vi "Main Page.vi"(8 "error in (no error)":errorcluster, 11 "Node Ptr":T3 format="%.0x") -> (0 "error out":errorcluster)   [LabVIEW 2023, in "Embedded TDMS Logger System Explorer.lvlib"]
uses:
  Embedded TDMS Logger System Explorer.lvlib
  <vilib>/NI VeriStand/Custom Device API/Custom Device Item Ref.ctl
  Shared/SegmentOptions.ctl
  <vilib>/NI VeriStand/Custom Device API/Custom Device Channel.ctl
  <vilib>/NI VeriStand/Custom Device API/Custom Device Channel Type.ctl
  Shared/Meta Data Item.ctl
  <vilib>/NI VeriStand/Custom Device API/Get Item Property (U16).vi
  <vilib>/NI VeriStand/Custom Device API/Get Item Property (String).vi
  <vilib>/NI VeriStand/Custom Device API/Set Item Property (String).vi
  <vilib>/NI VeriStand/Custom Device API/Set Item Property (U16).vi
  <vilib>/NI VeriStand/Custom Device API/Get Item Property (Variant).vi
  <vilib>/NI VeriStand/Custom Device API/Set Item Property (Variant).vi
  <vilib>/NI VeriStand/Custom Device API/Set Item Property (Boolean).vi
  <vilib>/NI VeriStand/Custom Device API/Set Item Property (U64).vi
  <vilib>/NI VeriStand/Custom Device API/Custom Device API.lvlib
  Shared/Embedded TDMS Logger Shared.lvlib
panel:
  in  "Tab Control":T1(tab)
  out "String 3":string="The data format can be specified in the string, as with the formats specified in: https://www.ni.com/docs/en-US/bundle/labview-api-ref/page/functions/format-date-time-string.html"
  in  "Segment every":dbl=3600.0
  in  "Segment by":T2=enum."Size (MB)"
  in  "Filename Format:":string="mytestfile_%Y-%M-%d-%H-%I-%S.tdms"
  in  "Log Directory":path=path "c:/nirt/veristand/logs"
  in  "Segment Files":bool=TRUE
  out "String":string="Unless set, the system will trigger immediately to log upon deployment. If triggering is however enabled the log will start when the trigger channel receives a non-zero value. It will only stop logging once the system is undeployed."
  in  "Start on Trigger":bool
  in  "File Level Meta Data":string[][](table)=[["Software Version"], ["Test Rig Used"], ["UUT"], ["Operator"]]
  in  "Async Timeout (ms)":u16
  out "Version":string
  in  "Specific Header":cluster{"Section Name":string}={"Section Name"="Custom Device Item Settings"}
  in  "General Header":cluster{"Section Name":string}={"Section Name"="General Custom Device Settings"}
  in  "Description":string
  in  "Name":string
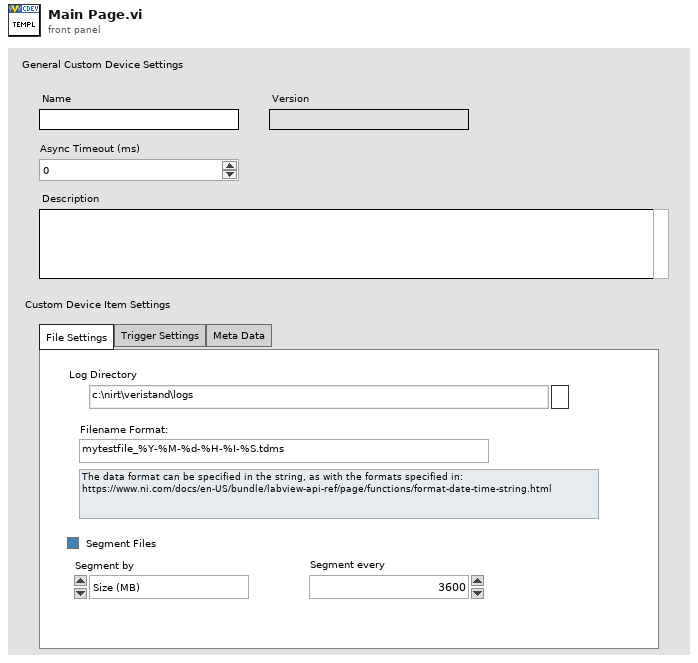
[diagram p1: front panel]
types:
  T1 = enum32{"File Settings", "Trigger Settings", "Meta Data"}
  T2 = typedef "SegmentOptions.ctl" = enum16{"Time (s)", "Size (MB)"}
  T3 = typedef "Custom Device API.lvlib/Custom Device Item Ref.ctl" = u64
  T4 = typedef "Custom Device API.lvlib/Custom Device Channel.ctl" = cluster{"Type":T5, "Units":string, "Default Value":dbl, "Faultable":bool, "Scalable":bool}
  T5 = typedef "Custom Device API.lvlib/Custom Device Channel Type.ctl" = enum16{"Input", "Output"}
  T6 = typedef "Custom Device API.lvlib/Custom Device Item Info.ctl" = cluster{"Name":string, "Is Channel":bool, "GUID":string, "Is Waveform":bool}
  T7 = typedef "Embedded TDMS Logger Shared.lvlib/Meta Data Item.ctl" = cluster{"Key":string, "Value":string}
  T8 = typedef "Custom Device API.lvlib/Custom Device Commands.ctl" = enum16{"Default", "Item renamed", "Shutdown", "Dynamic button pressed"}
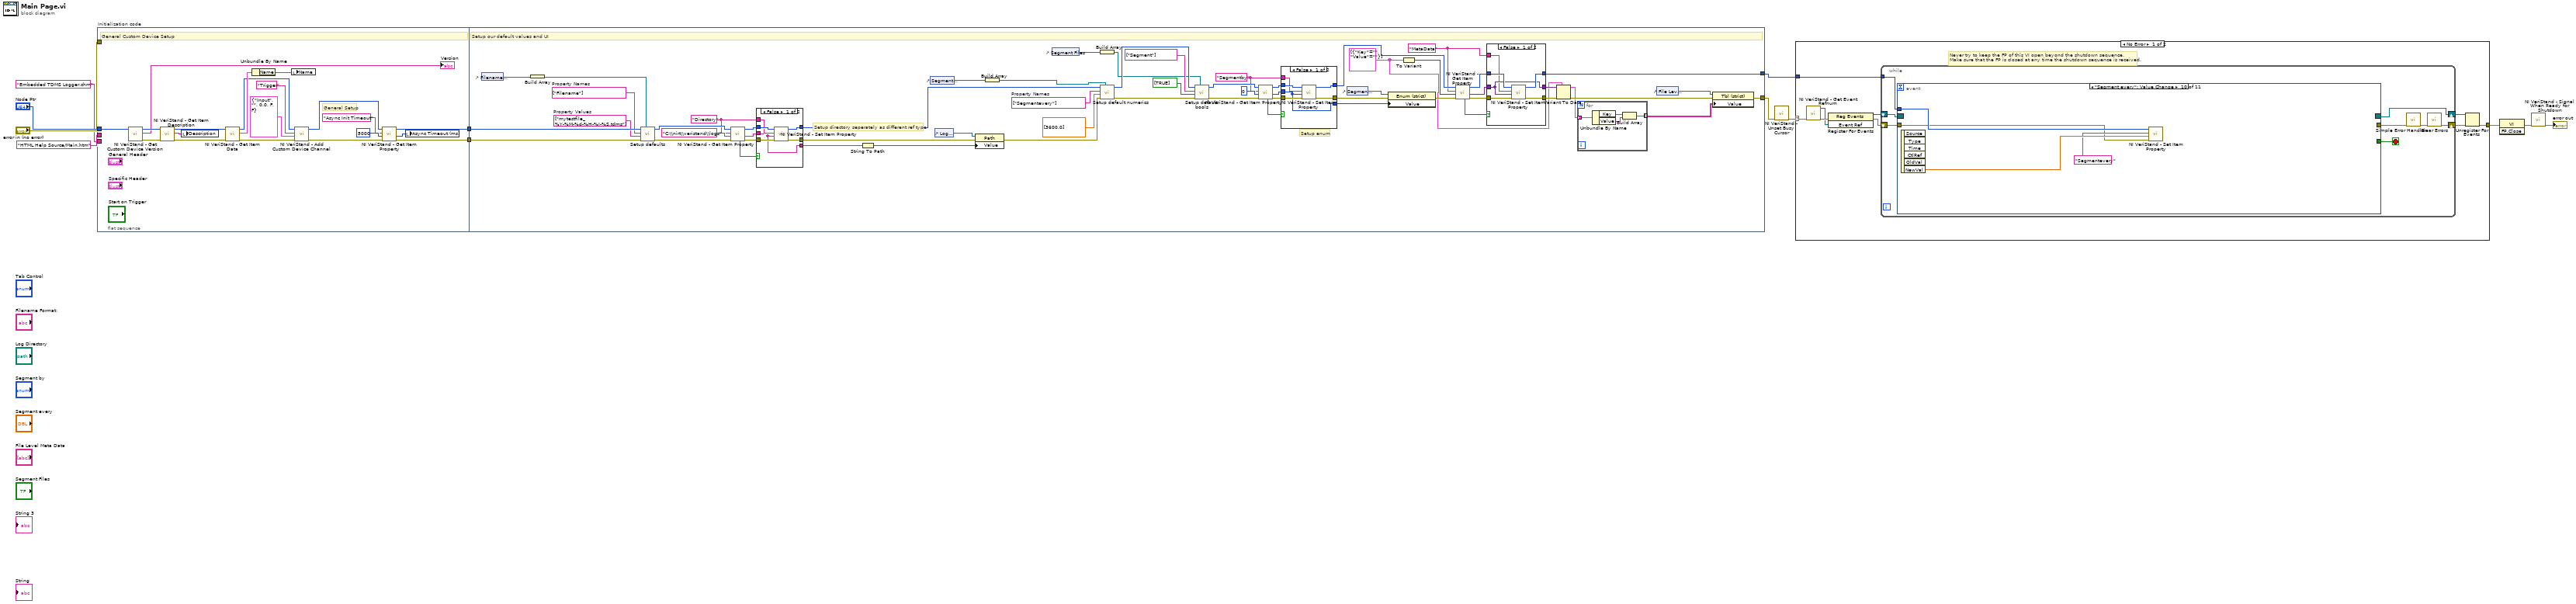
[diagram p0: block diagram]
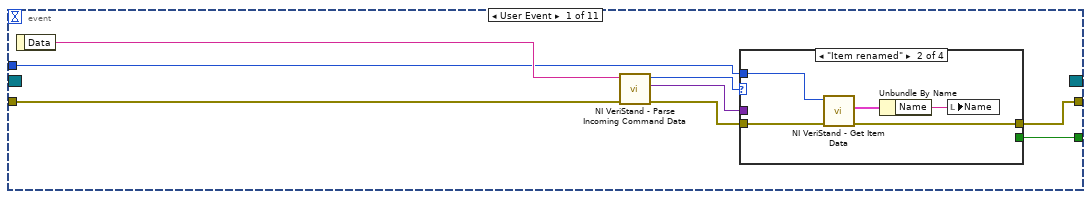
[diagram p2: hidden frame]
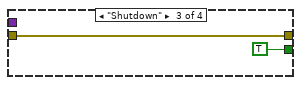
[diagram p4: hidden frame]
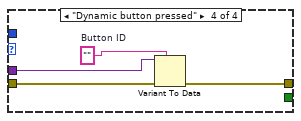
[diagram p5: hidden frame]
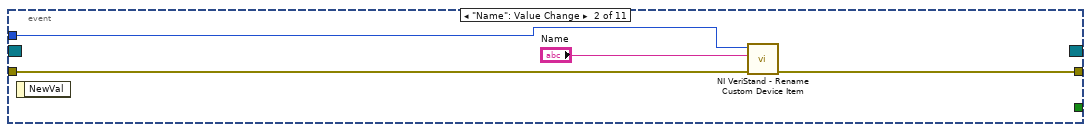
[diagram p6: hidden frame]
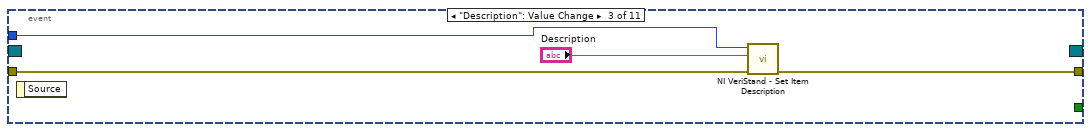
[diagram p7: hidden frame]
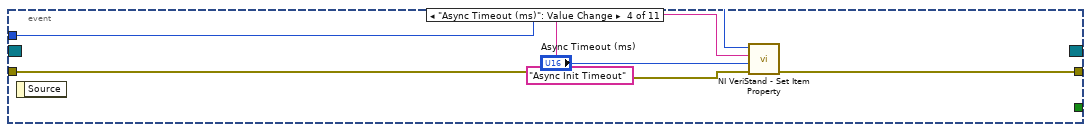
[diagram p8: hidden frame]
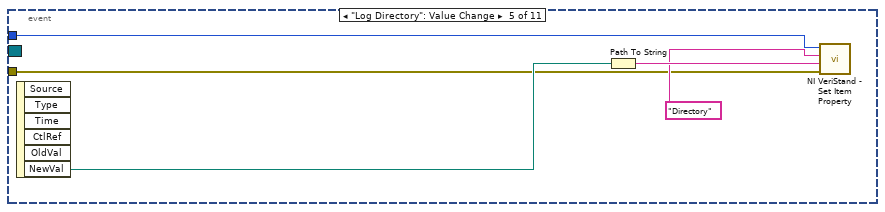
[diagram p9: hidden frame]
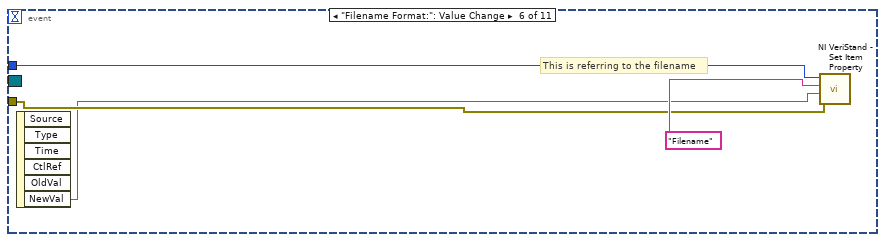
[diagram p10: hidden frame]
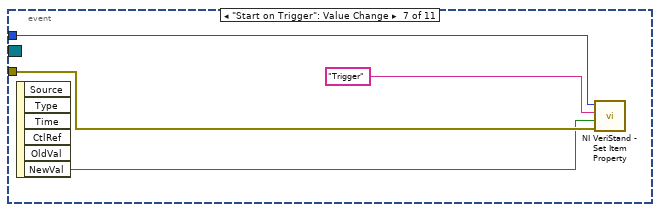
[diagram p11: hidden frame]
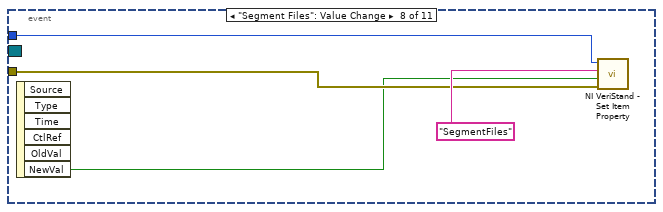
[diagram p12: hidden frame]
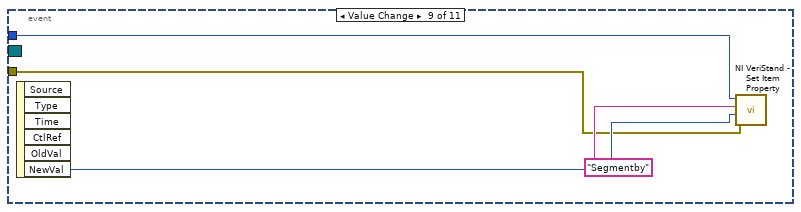
[diagram p13: hidden frame]
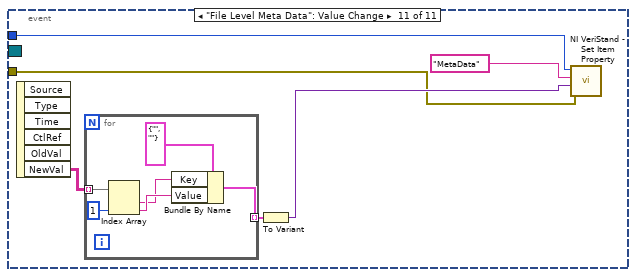
[diagram p14: hidden frame]
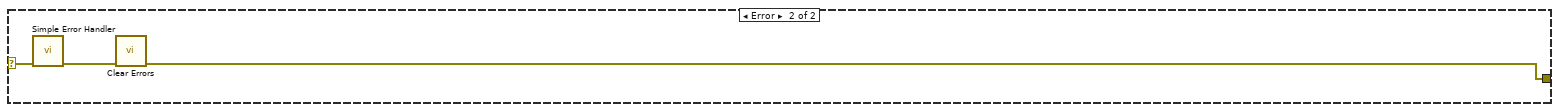
[diagram p15: hidden frame]
diagram:
  n1 = flat-sequence "Initialization code" {
    tunnel: "error in (no error)" -> [_]
    tunnel: "Node Ptr" -> [w29]
    tunnel: "HTML Help Source/Main.htm" ("HTML File") -> [_]
    tunnel: "Embedded TDMS Logger.chm" ("CD_CHM_FileName") -> [_]
    tunnel: [w14] -> w4
    tunnel: [w13] -> w3
    tunnel: w4 -> [w90]
    tunnel: w3 -> [w89]
    tunnel: [w43] -> w2
    tunnel: [w42] -> w1
    frame #0 {
      # "General Setup"
      # "General Custom Device Setup"
      n2 = call <vilib>:"NI VeriStand - Get Custom Device Version.vi"("Device Ref in"=w29) -> ("error out"=w28:errorcluster, "Value"=→"Version":string, "Device Ref out"=w27:T3)  [unwired: 8 in]
      n3 = call <vilib>:"NI VeriStand - Get Item Description.vi"("error in (no error)"=w28, "Item Ref in"=w27) -> ("error out"=w31:errorcluster, "Description"=w24:string, "Item Ref out"=w32:T3)  [unwired: 7 out]
      n4 = local write "Description"(w24) -> ()
      n5 = call <vilib>:"NI VeriStand - Get Item Data.vi"("error in (no error)"=w31, "Item Ref in"=w32) -> ("error out"=w19:errorcluster, "Item Info"=w30:T6, "Item Ref out"=w20:T3)  [unwired: 7 out]
      n6 = Unbundle By Name(w30) -> ("Name"=w25:string)
      n7 = local write "Name"(w25) -> ()
      n8 = call <vilib>:"NI VeriStand - Add Custom Device Channel.vi"("error in (no error)"=w19, "Channel"=T4 {"Type"=enum."Input", "Units"="", "Default Value"=0.0, "Faultable"=FALSE, "Scalable"=FALSE}, "Channel Name"="Trigger", "Parent Ref in"=w20) -> ("error out"=w16:errorcluster, "Parent Ref out"=w15:T3)  [unwired: 4 in, 2 out]
      n9 = call-poly <vilib>:"NI VeriStand - Get Item Property.vi"("error in (no error)"=w16, "Default Value"=u16 5000, "Property Name"="Async Init Timeout", "Item Ref in"=w15) -> ("error out"=w14:errorcluster, "Value"=w23:u16, "Item Ref out"=w13:T3)  [unwired: 4 in, 1 out]
      n10 = local write "Async Timeout (ms)"(w23) -> ()
    }
    frame #1 {
      w33 = T7[] [{"Key"="", "Value"=""}]
      w40 = "MetaData" ("Property Name")
      w50 = "Segmentby"
      w70 = string[] ["Segmentevery"]  # Property Names
      w75 = "Directory"
      w77 = string[] ["mytestfile_%Y-%M-%d-%H-%I-%S.tdms"]  # Property Values
      w88 = string[] ["Filename"]  # Property Names
      # "Setup enum"
      # "Setup directory seperately as different ref type"
      # "Setup our default values and UI"
      n11 = control-ref of="Filename Format:"() -> (w86:refnum<vi>)
      n12 = Build Array(w86) -> (w87:refnum<vi>[])
      n13 = call "Setup defaults.vi"("References"=w87, "error in (no error)"=w90, "Property Values"=w77, "Property Names"=w88, "Item Ref In"=w89) -> ("error out"=w79:errorcluster, "Item Ref out"=w78:T3)  [unwired: 5 in]
      n14 = call-poly <vilib>:"NI VeriStand - Get Item Property.vi"("error in (no error)"=w79, "Default Value"="C:\\nirt\\veristand\\logs", "Property Name"=w75, "Item Ref in"=w78) -> ("error out"=w83:errorcluster, "Value"=w81:string, "Item Ref out"=w82:T3, "Found?"=w84:bool)  [unwired: 4 in]
      n15 = case shown="False" w84 {
        tunnel: [w118 w121] -> w67
        tunnel: w82 -> [w117 w121]
        tunnel: [w116 w120] -> w85
        tunnel: w83 -> [w115 w120]
        tunnel: w81 -> [w113 w119]
        tunnel: [w113 w119] -> w73
        tunnel: w75 -> [w114 _]
        frame False {
          n16 = call-poly <vilib>:"NI VeriStand - Set Item Property.vi"("error in (no error)"=w115, "Value"=w113, "Property Name"=w114, "Item Ref in"=w117) -> ("error out"=w116:errorcluster, "Item Ref out"=w118:T3)  [unwired: 5 in, 1 out]
        }
        frame True {
        }
      }
      n17 = String To Path(string=w73) -> (path=w74:path)
      n18 = control-ref of="Segment every"() -> (w72:refnum<vi>)
      n19 = control-ref of="Log Directory"() -> (w80:refnum<vi>)
      n20 = property class="Path"(reference=w80, error in=w85, "Value"=w74) -> (error out=w65:errorcluster)  [unwired: 1 out]
      n21 = Build Array(w72) -> (w68:refnum<vi>[])
      n22 = control-ref of="Segment Files"() -> (w71:refnum<vi>)
      n23 = Build Array(w71) -> (w61:refnum<vi>[])
      n24 = call "Setup default numerics.vi"("References"=w68, "error in (no error)"=w65, "Property Values"=dbl[] [3600.0], "Property Names"=w70, "Item Ref In"=w67) -> ("error out"=w64:errorcluster, "Item Ref out"=w66:T3)  [unwired: 5 in]
      n25 = call "Setup default bools.vi"("appended array"=w61, "error in (no error)"=w64, "Property Values"=bool[] [TRUE], "Property Names"=string[] ["Segment"], "Item Ref In"=w66) -> ("error out"=w55:errorcluster, "Item Ref out"=w54:T3)  [unwired: 5 in]
      n26 = call-poly <vilib>:"NI VeriStand - Get Item Property.vi"("error in (no error)"=w55, "Default Value"=u16 0, "Property Name"=w50, "Item Ref in"=w54) -> ("error out"=w58:errorcluster, "Value"=w60:u16, "Item Ref out"=w59:T3, "Found?"=w57:bool)  [unwired: 4 in]
      n27 = case shown="False" w57 {
        tunnel: [w109 w112] -> w45
        tunnel: w59 -> [w108 w112]
        tunnel: [w107 w111] -> w56
        tunnel: w58 -> [w106 w111]
        tunnel: w60 -> [w105 w110]
        tunnel: [w105 w110] -> w51
        tunnel: w50 -> [w104 _]
        frame False {
          n28 = call-poly <vilib>:"NI VeriStand - Set Item Property.vi"("error in (no error)"=w106, "Value"=w105, "Property Name"=w104, "Item Ref in"=w108) -> ("error out"=w107:errorcluster, "Item Ref out"=w109:T3)  [unwired: 5 in, 1 out]
        }
        frame True {
        }
      }
      n29 = control-ref of="Segment by"() -> (w53:refnum<vi>)
      n30 = property class="Enum (strict)"(reference=w53, error in=w56, "Value"=w51) -> (error out=w41:errorcluster)  [unwired: 1 out]
      n31 = To Variant(anything=w33) -> (Variant=w46:variant)
      n32 = call-poly <vilib>:"NI VeriStand - Get Item Property.vi"("error in (no error)"=w41, "Default Value"=w46, "Property Name"=w40, "Item Ref in"=w45) -> ("error out"=w48:errorcluster, "Value"=w47:variant, "Item Ref out"=w44:T3, "Found?"=w49:bool)  [unwired: 4 in]
      n33 = case shown="False" w49 {
        tunnel: [w100 w103] -> w43
        tunnel: w44 -> [w99 w103]
        tunnel: [w98 w102] -> w38
        tunnel: w48 -> [w97 w102]
        tunnel: w47 -> [w96 w101]
        tunnel: [w96 w101] -> w36
        tunnel: w40 -> [w95 _]
        frame False {
          n34 = call-poly <vilib>:"NI VeriStand - Set Item Property.vi"("error in (no error)"=w97, "Value"=w96, "Property Name"=w95, "Item Ref in"=w99) -> ("error out"=w98:errorcluster, "Item Ref out"=w100:T3)  [unwired: 5 in, 1 out]
        }
        frame True {
        }
      }
      n35 = Variant To Data(error in=w38, type=w33, Variant=w36) -> (data=w34:T7[], error out=w37:errorcluster)
      n36 = for {
        tunnel: [w92] -> w35 mode=indexing
        tunnel: w34 -> [w91] mode=indexing
        n37 = Unbundle By Name(w91) -> ("Key"=w94:string, "Value"=w93:string)
        n38 = Build Array(w94, w93) -> (w92:string[])
      }
      n39 = control-ref of="File Level Meta Data"() -> (w39:refnum<vi>)
      n40 = property class="Tbl (strict)"(reference=w39, error in=w37, "Value"=w35) -> (error out=w42:errorcluster)  [unwired: 1 out]
    }
  }
  n41 = call <vilib>:"NI VeriStand - Unset Busy Cursor.vi"("error in (no error)"=w1) -> ("error out"=w8:errorcluster)  [unwired: 10 out]
  n42 = case shown="No Error" w8 {
    selector: w8 -> [w123 w211]
    tunnel: [w127 w209] -> w12
    tunnel: w2 -> [w122 _]
    frame No Error {
      # "Never try to keep the FP of this VI open beyond the shutdown sequence.\nMake sure that the FP is closed at any time the shutdown sequence is received."
      n43 = call <vilib>:"NI VeriStand - Get Event Refnum.vi"("error in (no error)"=w123) -> ("error out"=w130:errorcluster, "Event Ref"=w126:refnum<user-event>)  [unwired: 9 out]
      n44 = register-events(error in=w130, w126) -> (reference out=w124:refnum<event-registration>, error out=w125:errorcluster)  [unwired: 1 in]
      n45 = while {
        shift-right: [w132] -> w128
        shift-left: w125 -> [w137]
        shift-right: [w138] -> w129
        shift-left: w124 -> [w136]
        tunnel: w122 -> [w131]
        stop <- w135 stop-if-true
        n46 = event shown="[9] \"Segment every\": Value Change" {
          selector: w136 -> [_ _ _ _ _ _ _ _ _ _ _]
          dyn-events: [_ _ _ _ _ _ _ _ _ _ _] -> w138
          timeout: _ -> [_ _ _ _ _ _ _ _ _ _ _]
          tunnel: w137 -> [w146 w162 w166 w171 w173 w179 w182 w187 w189 w193 w199]
          tunnel: [w142 _ _ _ _ _ _ _ _ _ _] -> w135
          tunnel: [w141 w161 w165 w169 _ _ _ _ _ _ _] -> w134
          tunnel: w131 -> [w139 w159 w163 w167 w172 w177 w183 w186 w190 w195 w200]
          event User Event {
            n47 = event-data() -> ("Data"=w145:string)  [unwired: 1 out]
            n48 = call <vilib>:"NI VeriStand - Parse Incoming Command Data.vi"("error in (no error)"=w146, "Incoming data"=w145) -> ("error out"=w144:errorcluster, "Outgoing data"=w140:variant, "Action"=w143:T8)  [unwired: 7 out]
            n49 = case shown="\"Item renamed\"" w143 {
              tunnel: w144 -> [w147 w152 w153 w158]
              tunnel: [_ _ TRUE _] -> w142
              tunnel: [w147 w150 w153 w155] -> w141
              tunnel: w140 -> [_ _ _ w157]
              tunnel: w139 -> [_ w148 _ _]
              frame "Default", Default {
              }
              frame "Item renamed" {
                n50 = call <vilib>:"NI VeriStand - Get Item Data.vi"("error in (no error)"=w152, "Item Ref in"=w148) -> ("error out"=w150:errorcluster, "Item Info"=w151:T6)  [unwired: 8 out]
                n51 = Unbundle By Name(w151) -> ("Name"=w149:string)
                n52 = local write "Name"(w149) -> ()
              }
              frame "Shutdown" {
              }
              frame "Dynamic button pressed" {
                w156 = ""  # Button ID
                n53 = Variant To Data(error in=w158, type=w156, Variant=w157) -> (error out=w155:errorcluster)  [unwired: 1 out]
              }
            }
          }
          event "Name": Value Change {
            n54 = event-data() -> ()  [unwired: 2 out]
            n55 = call <vilib>:"NI VeriStand - Rename Custom Device Item.vi"("error in (no error)"=w162, "New Name"="Name", "Item Ref in"=w159) -> ("error out"=w161:errorcluster)  [unwired: 1 in, 7 out]
          }
          event "Description": Value Change {
            n56 = event-data() -> ()  [unwired: 2 out]
            n57 = call <vilib>:"NI VeriStand - Set Item Description.vi"("error in (no error)"=w166, "Description"="Description", "Item Ref in"=w163) -> ("error out"=w165:errorcluster)  [unwired: 8 out]
          }
          event "Async Timeout (ms)": Value Change {
            n58 = event-data() -> ()  [unwired: 2 out]
            n59 = call-poly <vilib>:"NI VeriStand - Set Item Property.vi"("error in (no error)"=w171, "Value"="Async Timeout (ms)", "Property Name"="Async Init Timeout", "Item Ref in"=w167) -> ("error out"=w169:errorcluster)  [unwired: 5 in, 2 out]
          }
          event "Log Directory": Value Change {
            n60 = event-data() -> ("NewVal"=w176:path)  [unwired: 6 out]
            n61 = Path To String(path=w176) -> (string=w175:string)
            n62 = call-poly <vilib>:"NI VeriStand - Set Item Property.vi"("error in (no error)"=w173, "Value"=w175, "Property Name"="Directory", "Item Ref in"=w172) -> ()  [unwired: 5 in, 3 out]
          }
          event "Filename Format:": Value Change {
            # "This is referring to the filename"
            n63 = event-data() -> ("NewVal"=w178:string)  [unwired: 6 out]
            n64 = call-poly <vilib>:"NI VeriStand - Set Item Property.vi"("error in (no error)"=w179, "Value"=w178, "Property Name"="Filename", "Item Ref in"=w177) -> ()  [unwired: 5 in, 3 out]
          }
          event "Start on Trigger": Value Change {
            n65 = event-data() -> ("NewVal"=w181:bool)  [unwired: 6 out]
            n66 = call-poly <vilib>:"NI VeriStand - Set Item Property.vi"("error in (no error)"=w182, "Value"=w181, "Property Name"="Trigger", "Item Ref in"=w183) -> ()  [unwired: 5 in, 3 out]
          }
          event "Segment Files": Value Change {
            n67 = event-data() -> ("NewVal"=w185:bool)  [unwired: 6 out]
            n68 = call-poly <vilib>:"NI VeriStand - Set Item Property.vi"("error in (no error)"=w187, "Value"=w185, "Property Name"="SegmentFiles", "Item Ref in"=w186) -> ()  [unwired: 5 in, 3 out]
          }
          event Value Change {
            n69 = event-data() -> ("NewVal"=w191:T2)  [unwired: 6 out]
            n70 = call-poly <vilib>:"NI VeriStand - Set Item Property.vi"("error in (no error)"=w189, "Value"=w191, "Property Name"="Segmentby", "Item Ref in"=w190) -> ()  [unwired: 5 in, 3 out]
          }
          event "Segment every": Value Change {
            n71 = event-data() -> ("NewVal"=w196:dbl)  [unwired: 6 out]
            n72 = call-poly <vilib>:"NI VeriStand - Set Item Property.vi"("error in (no error)"=w193, "Value"=w196, "Property Name"="Segmentevery", "Item Ref in"=w195) -> ()  [unwired: 5 in, 3 out]
          }
          event "File Level Meta Data": Value Change {
            n73 = event-data() -> ("NewVal"=w197:string[][])  [unwired: 6 out]
            n74 = for {
              tunnel: [w207] -> w198 mode=indexing
              tunnel: w197 -> [w203] mode=indexing
              n75 = Index Array(array=w203, index #2=1 ("index")) -> (element #1=w204:string, element #2=w205:string)  [unwired: 1 in]
              n76 = Bundle By Name(cluster=T7 {"Key"="", "Value"=""} ("Meta Data"), "Key"=w204, "Value"=w205) -> (w207:T7)
            }
            n77 = To Variant(anything=w198) -> (Variant=w202:variant)
            n78 = call-poly <vilib>:"NI VeriStand - Set Item Property.vi"("error in (no error)"=w199, "Value"=w202, "Property Name"="MetaData", "Item Ref in"=w200) -> ()  [unwired: 5 in, 3 out]
          }
        }
        n79 = call <vilib>:"Simple Error Handler.vi"("error in (no error)"=w134) -> ("error out"=w133:errorcluster)  [unwired: 1 in, 7 out]
        n80 = call <vilib>:"Clear Errors.vi"("error in (no error)"=w133) -> ("error out"=w132:errorcluster)  [unwired: 1 in, 5 out]
      }
      n81 = Unregister For Events(event registration refnum=w129, error in=w128) -> (error out=w127:errorcluster)
    }
    frame Error {
      n82 = call <vilib>:"Simple Error Handler.vi"("error in (no error)"=w211) -> ("error out"=w210:errorcluster)  [unwired: 1 in, 7 out]
      n83 = call <vilib>:"Clear Errors.vi"("error in (no error)"=w210) -> ("error out"=w209:errorcluster)  [unwired: 1 in, 5 out]
    }
  }
  n84 = invoke class="VI" method="FP.Close"(error in=w12) -> (error out=w11:errorcluster)  [unwired: 2 in, 2 out]
  n85 = call <vilib>:"NI VeriStand - Signal When Ready for Shutdown.vi"("error in (no error)"=w11) -> ("error out"=→"error out":errorcluster)  [unwired: 10 out]
